vi "Update Display.vi"(8 "error in (no error)":errorcluster, 11 "Spanish Picker in":refnum<class "Spanish Picker.lvclass">) -> (0 "error out":errorcluster, 3 "Spanish Picker out":refnum<class "Spanish Picker.lvclass">)   [LabVIEW 2020, in "Spanish Picker.lvlib" / "Spanish Picker.lvclass"]
uses:
  Spanish Picker.lvclass
  Spanish Picker.lvclass/Spanish Picker.ctl
  Products Picker/Products Picker.lvclass
  D:/Storage/Source Code/Clase AF/ClaseAF/05 AF Camera/Products Picker/Products Picker.lvclass
  C:/Program Files (x86)/National Instruments/LabVIEW 2020/vi.lib/ActorFramework/Actor/Actor.lvclass
  D:/Storage/Source Code/Clase AF/ClaseAF/05 AF Camera/Spanish Picker/Spanish Picker.lvclass
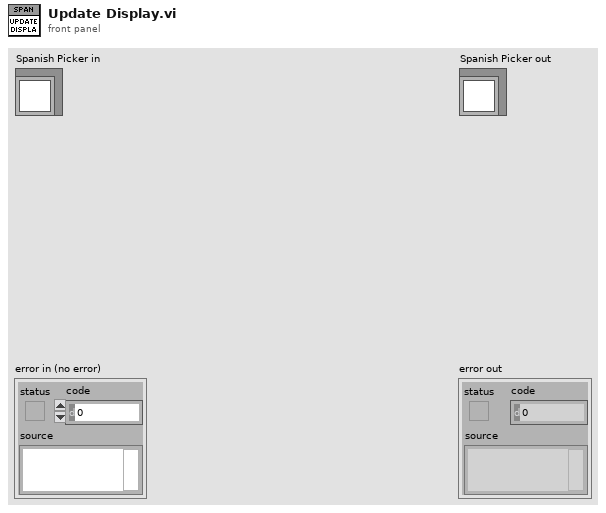
[diagram p1: front panel]
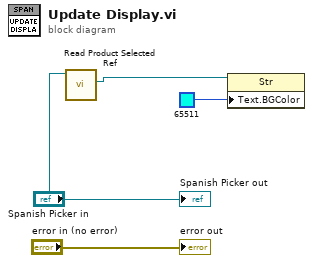
[diagram p0: block diagram]
diagram:
  n1 = call "Read Product Selected Ref.vi"("Products Picker in"="Spanish Picker in") -> ("Product Selected Ref"=w2:refnum<vi>)  [unwired: 9 in, 1 out]
  n2 = property on="Property Node" class="Str"(reference=w2, "Text.BGColor"=u32 65511) -> ()  [unwired: 1 in, 2 out]
  "error out" <- "error in (no error)"
  "Spanish Picker out" <- "Spanish Picker in"
